vi "Model Analysis Main.vi"(8 "error in (no error)":errorcluster, 10 "Current Path":string, 11 "SDF Ref":refnum<k24>) -> (0 "error out":errorcluster)   [LabVIEW 2016, in "System Mapping Tool.lvlib"]
uses:
  System Mapping Tool.lvlib
  NationalInstruments.VeriStand.SystemStorageUI
  NationalInstruments.VeriStand.SystemDefinitionAPI
  TypeDefs/Model Analysis Data.ctl
  TypeDefs/Model Analysis UI Refs.ctl
panel:
  out "Model Signal Count":i32
  out "Model Parameter Count":i32
  out "Model Outport Count":i32
  out "Model Inport Count":i32
  in  "Key":i32(listbox)
  in  "Analyze Parameter File":bool
  in  "Model Signals":i32(listbox)
  in  "Model Parameters":i32(listbox)
  in  "Model Outports":i32(listbox)
  in  "Model Inports":i32(listbox)
  in  "Refresh":bool
  in  "Model Path":string
  in  "Model Name":string
  in  "TreeAliasBrowserWF":refnum<k24>(container)
  in  "OK":bool
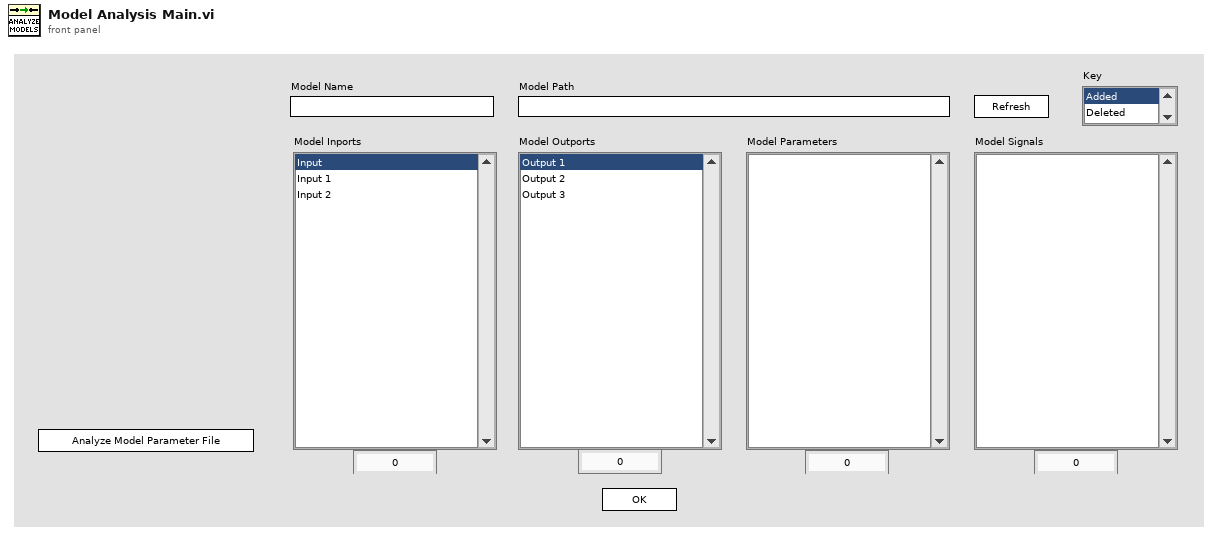
[diagram p1: front panel]
types:
  T1 = enum8{"Enabled", "Disabled", "Disabled and Grayed Out"}
  T2 = typedef "System Mapping Tool.lvlib/Model Analysis UI Refs.ctl" = cluster{"Tree Ref":refnum<k24>, "Model Name Ref":refnum<vi>, "Model Path Ref":refnum<vi>, "Model Inports Ref":refnum<vi>, "Model Outports Ref":refnum<vi>, "Model Parameters Ref":refnum<vi>, "Model Signals Ref":refnum<vi>, "Refresh Ref":refnum<vi>, "Analyze Parameter File Ref":refnum<vi>, "Model Inport Count Ref":refnum<vi>, "Model Outport Count Ref":refnum<vi>, "Model Parameter Count Ref":refnum<vi>, "Model Signal Count Ref":refnum<vi>}
  T3 = typedef "System Mapping Tool.lvlib/Model Analysis Data.ctl" = cluster{"UI Refs":T2, "SDF Ref":refnum<k24>, "Current Model Path":string}
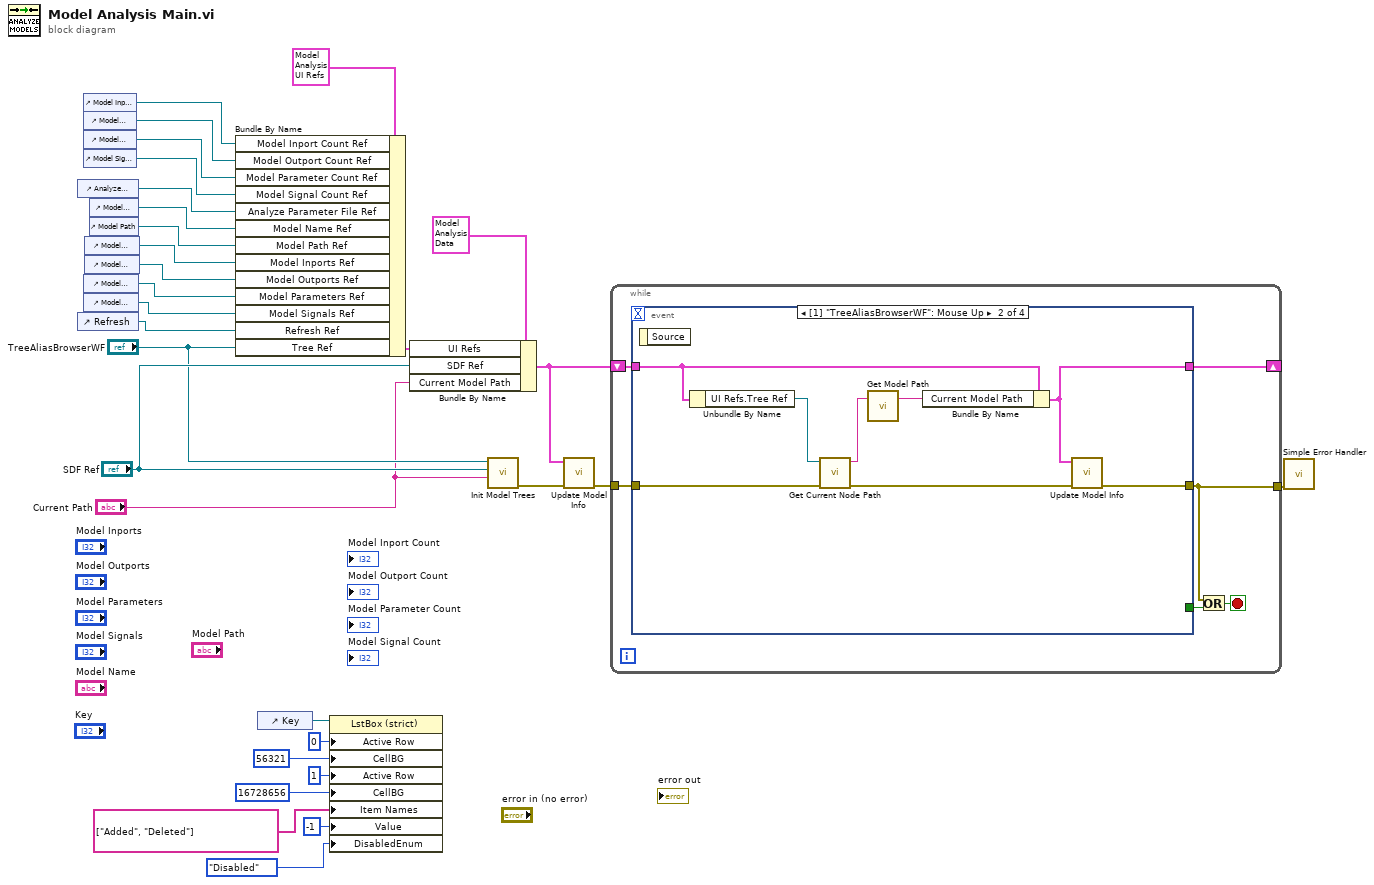
[diagram p0: block diagram]
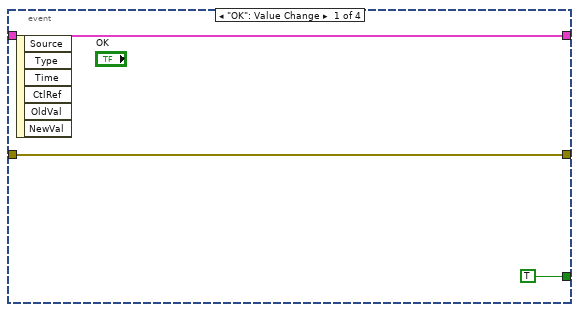
[diagram p2: hidden frame]
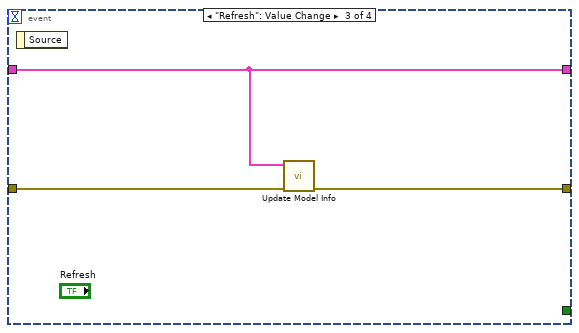
[diagram p3: hidden frame]
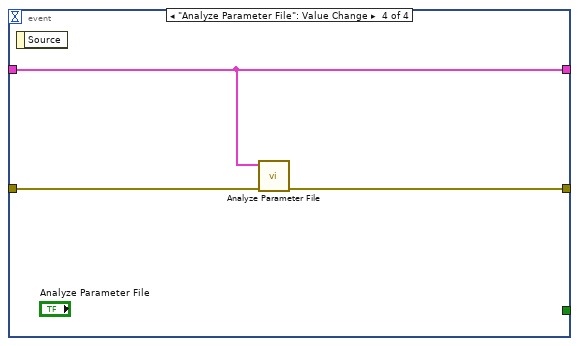
[diagram p4: hidden frame]
diagram:
  n1 = control-ref of="Analyze Parameter File"() -> (w5:refnum<vi>)
  n2 = control-ref of="Refresh"() -> (w24:refnum<vi>)
  n3 = control-ref of="Model Inport Count"() -> (w4:refnum<vi>)
  n4 = control-ref of="Model Outport Count"() -> (w3:refnum<vi>)
  n5 = control-ref of="Model Parameter Count"() -> (w2:refnum<vi>)
  n6 = control-ref of="Model Signal Count"() -> (w1:refnum<vi>)
  n7 = control-ref of="Model Parameters"() -> (w15:refnum<vi>)
  n8 = control-ref of="Model Signals"() -> (w14:refnum<vi>)
  n9 = control-ref of="Model Inports"() -> (w17:refnum<vi>)
  n10 = control-ref of="Model Outports"() -> (w16:refnum<vi>)
  n11 = control-ref of="Model Name"() -> (w23:refnum<vi>)
  n12 = control-ref of="Model Path"() -> (w22:refnum<vi>)
  n13 = Bundle By Name(cluster=T2 {"Tree Ref"=refnum, "Model Name Ref"=refnum, "Model Path Ref"=refnum, "Model Inports Ref"=refnum, "Model Outports Ref"=refnum, "Model Parameters Ref"=refnum, "Model Signals Ref"=refnum, "Refresh Ref"=refnum, "Analyze Parameter File Ref"=refnum, "Model Inport Count Ref"=refnum, "Model Outport Count Ref"=refnum, "Model Parameter Count Ref"=refnum, "Model Signal Count Ref"=refnum} ("UI Refs"), "Model Inport Count Ref"=w4, "Model Outport Count Ref"=w3, "Model Parameter Count Ref"=w2, "Model Signal Count Ref"=w1, "Analyze Parameter File Ref"=w5, "Model Name Ref"=w23, "Model Path Ref"=w22, "Model Inports Ref"=w17, "Model Outports Ref"=w16, "Model Parameters Ref"=w15, "Model Signals Ref"=w14, "Refresh Ref"=w24, "Tree Ref"="TreeAliasBrowserWF") -> (w25:T2)
  n14 = control-ref of="Key"() -> (w13:refnum<vi>)
  n15 = property class="LstBox (strict)"(reference=w13, "Active Row"=0 ("Active Row:Active Row Number"), "CellBG"=u32 56321 ("Active Row:Cell Background Color"), "Active Row"=1 ("Active Row:Active Row Number"), "CellBG"=u32 16728656 ("Active Row:Cell Background Color"), "Item Names"=string[] ["Added", "Deleted"], "Value"=-1 ("Active Row:Active Row Number"), "DisabledEnum"=T1."Disabled" ("Disabled")) -> ()  [unwired: 1 in, 2 out]
  n16 = Bundle By Name(cluster=T3 {"UI Refs"={"Tree Ref"=refnum, "Model Name Ref"=refnum, "Model Path Ref"=refnum, "Model Inports Ref"=refnum, "Model Outports Ref"=refnum, "Model Parameters Ref"=refnum, "Model Signals Ref"=refnum, "Refresh Ref"=refnum, "Analyze Parameter File Ref"=refnum, "Model Inport Count Ref"=refnum, "Model Outport Count Ref"=refnum, "Model Parameter Count Ref"=refnum, "Model Signal Count Ref"=refnum}, "SDF Ref"=refnum, "Current Model Path"=""} ("Loop Data"), "UI Refs"=w25, "SDF Ref"="SDF Ref", "Current Model Path"="Current Path") -> (w19:T3)
  n17 = call "Init Model Trees.vi"("Model to Highlight"="Current Path", "SDF Ref"="SDF Ref", "Tree Ref"="TreeAliasBrowserWF") -> ("error out"=w21:errorcluster)  [unwired: 8 in]
  n18 = call "Update Model Info.vi"("error in (no error)"=w21, "Loop Data"=w19) -> ("error out"=w20:errorcluster)  [unwired: 9 in]
  n19 = while {
    tunnel: w20 -> [w36]
    tunnel: [w33] -> w30
    shift-right: [w31] -> _
    shift-left: w19 -> [w32]
    stop <- w34 stop-if-true
    n20 = event shown="[1] \"TreeAliasBrowserWF\": Mouse Up" {
      selector: _ -> [_ _ _ _]
      dyn-events: _ -> [_ _ _ _]
      timeout: _ -> [_ _ _ _]
      tunnel: w36 -> [w38 w47 w50 w53]
      tunnel: [TRUE _ _ _] -> w35
      tunnel: [w38 w40 w48 w52] -> w33
      tunnel: w32 -> [w37 w44 w49 w51]
      tunnel: [w37 w42 w49 w51] -> w31
      event "OK": Value Change {
        n21 = event-data() -> ()  [unwired: 1 in, 6 out]
      }
      event "TreeAliasBrowserWF": Mouse Up {
        n22 = event-data() -> ()  [unwired: 1 in, 1 out]
        n23 = Unbundle By Name(w44) -> ("UI Refs.Tree Ref"=w46:refnum<k24>)
        n24 = call "Get Current Node Path.vi"("error in (no error)"=w47, "Tree Ref"=w46) -> ("error out"=w41:errorcluster, "Current Node Path"=w45:string)  [unwired: 8 in]
        n25 = call "Get Model Path.vi"("Node Path"=w45) -> ("Model Path"=w43:string)  [unwired: 2 in]
        n26 = Bundle By Name(cluster=w44, "Current Model Path"=w43) -> (w42:T3)
        n27 = call "Update Model Info.vi"("error in (no error)"=w41, "Loop Data"=w42) -> ("error out"=w40:errorcluster)  [unwired: 9 in]
      }
      event "Refresh": Value Change {
        n28 = event-data() -> ()  [unwired: 1 in, 1 out]
        n29 = call "Update Model Info.vi"("error in (no error)"=w50, "Loop Data"=w49) -> ("error out"=w48:errorcluster)  [unwired: 9 in]
      }
      event "Analyze Parameter File": Value Change {
        n30 = event-data() -> ()  [unwired: 1 in, 1 out]
        n31 = call "Analyze Parameter File.vi"("error in (no error)"=w53, "Loop Data"=w51) -> ("error out"=w52:errorcluster)  [unwired: 9 in]
      }
    }
    n32 = Or(x=w33, y=w35) -> (x .or. y?=w34:bool)
  }
  n33 = call <vilib>:"Simple Error Handler.vi"("error in (no error)"=w30) -> ()  [unwired: 4 in, 5 out]
